vi "SDCP FTOR Encode and Decode Test.vi"() -> ()   [LabVIEW 2020]
uses:
  Typedefs/SDCP FTOR params.ctl
panel:
  out "FTOR2 frame":u8[](array[numeric])
  out "FTOR1 frame":u8[](array[numeric])
  out "FTOR registers out":T1
  in  "FTOR registers in":T1
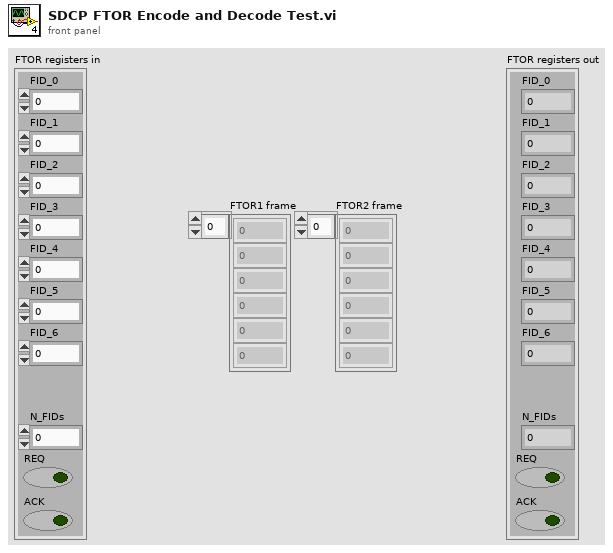
[diagram p1: front panel]
types:
  T1 = typedef "SDCP FTOR params.ctl" = cluster{"FID_0":i32, "FID_1":i32, "FID_2":i32, "FID_3":i32, "FID_4":i32, "FID_5":i32, "FID_6":i32, "N_FIDs":i32, "REQ":bool, "ACK":bool}
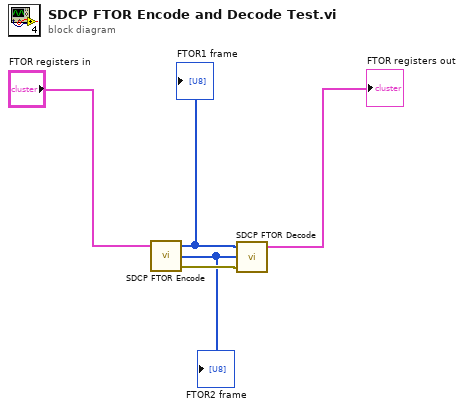
[diagram p0: block diagram]
diagram:
  n1 = call "SDCP FTOR Encode.vi"(5:"FTOR registers in") -> ("error out"=w4:errorcluster, "FTOR2 frame"=w2:u8[], "FTOR1 frame"=w3:u8[])  [unwired: 2 in]
  "FTOR1 frame" <- w3
  "FTOR2 frame" <- w2
  n2 = call "SDCP FTOR Decode.vi"("error in (no error)"=w4, "FTOR2 frame"=w2, "FTOR1 frame"=w3) -> ("out"=→"FTOR registers out":T1)  [unwired: 1 in, 1 out]
